vi "BtnColor.vi"(7 "Selector":dbl) -> (0 "Text Color":i32, 2 "Colors":cluster{u32, u32}[](array[cluster]), 3 "Text":string, 5 "Disabled":i32)   [LabVIEW 2016]
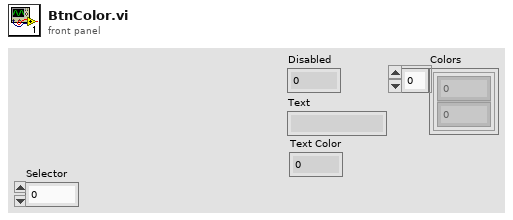
[diagram p1: front panel]
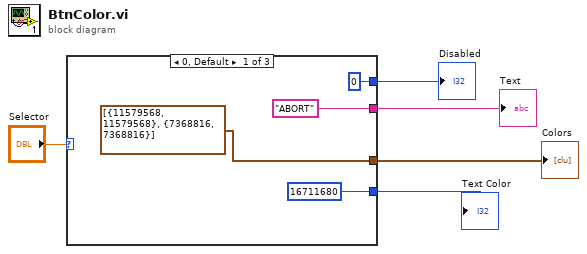
[diagram p0: block diagram]
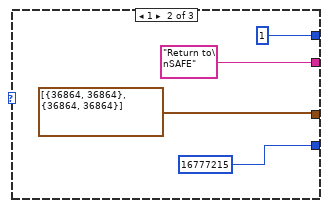
[diagram p2: hidden frame]
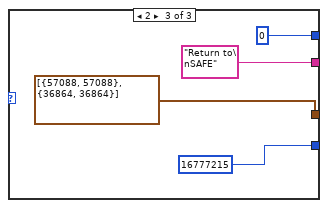
[diagram p3: hidden frame]
diagram:
  n1 = case shown="0, Default" "Selector" {
    tunnel: [0 1 0] -> w4
    tunnel: ["ABORT" "Return to\nSAFE" "Return to\nSAFE"] -> w1
    tunnel: [cluster{u32, u32}[] [{11579568, 11579568}, {7368816, 7368816}] ("Colors [4]") cluster{u32, u32}[] [{36864, 36864}, {36864, 36864}] ("Colors [4]") cluster{u32, u32}[] [{57088, 57088}, {36864, 36864}] ("Colors [4]")] -> w3
    tunnel: [16711680 16777215 16777215] -> w2
    frame 0, Default {
    }
    frame 1 {
    }
    frame 2 {
    }
  }
  "Disabled" <- w4
  "Text" <- w1
  "Colors" <- w3
  "Text Color" <- w2
